vi "Build Less Compare Types.vi"   [LabVIEW 2021]
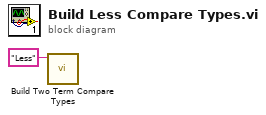
[diagram p0: block diagram]
diagram:
  n1 = call "Build Two Term Compare Types.vi"("Comparison Name"="Less") -> ()  [unwired: 11 in]
